vi "ReadData4.vi"() -> ()   [LabVIEW 2013]
uses:
  <vilib>/Utility/file.llb/Read From Spreadsheet File (DBL).vi
  <vilib>/Analysis/NI_AALPro.lvlib
  <vilib>/Analysis/NI_AALBase.lvlib
panel:
  out "Residual (V)":dbl=0.0015783758566444736 format="%#_3g"
  in  "1st sweep":i32=400
  out "Peak Area Distribution":cluster{"Y":dbl[], "Y":dbl[]}[](graph)
  in  "# of sweeps":i32=500
  out "Mean Error":dbl=-0.0 format="%#_2g"
  out "Mean Area":dbl=nan format="%#_4g"
  out "Peak Area":dbl(graph)=0.01758465336266432
  out "Spectrum #":i32=99
  out "Chars":i32=127116
  out "Fcen":dbl=213.0 format="%#_13g"
  out "Fmin":dbl=212.75 format="%#_13g"
  out "Fmax":dbl=213.25 format="%#_13g"
  out "# Data points":i32=101
  out "Peak Area (V-MHz)":dbl=0.01758465336266432 format="%#_3g"
  out "Offset V":dbl=0.15883666666666665 format="%#_3g"
  out "RMS Fit Error (V)":dbl=0.02098351608245331 format="%#_2g"
  in  "Start sigma (V)":dbl=0.01 format="%#_13g"
  in  "Start offset (V)":dbl format="%#_13g"
  out "FWHM (MHz)":dbl=0.06356226437922968 format="%#_3g"
  out "Center Freq (MHz)":dbl=213.00605703700742
  out "Amplitude (V)":dbl=0.2594313715946598 format="%#_3g"
  out "NMR Graph + Fit":cluster{cluster{dbl, "Numeric":dbl}[]}[](graph)=[{[{212.75, "Numeric"=0.0015783758566444736}, {212.755, "Numeric"=0.0015783758566444736}, {212.76, "Numeric"=0.0015783758566444738}, {212.765, "Numeric"=0.001578375856644475}, {212.77, "Numeric"=0.0015783758566444812}, {212.775, "Numeric"=0.0015783758566445105}, {212.78, "Numeric"=0.0015783758566446499}, {212.785, "Numeric"=0.0015783758566452857}, {212.79, "Numeric"=0.0015783758566480905}, {212.795, "Numeric"=0.0015783758566600408}, {212.8, "Numeric"=0.0015783758567092245}, {212.805, "Numeric"=0.001578375856904754}, {212.81, "Numeric"=0.0015783758576555789}, {212.815, "Numeric"=0.0015783758604403309}, {212.82, "Numeric"=0.0015783758704160137}, {212.825, "Numeric"=0.0015783759049296919}, {212.83, "Numeric"=0.0015783760202526297}, {212.835, "Numeric"=0.0015783763923853246}, {212.84, "Numeric"=0.0015783775520111368}, {212.845, "Numeric"=0.0015783810414393363}, {212.85, "Numeric"=0.001578391180165903}, {212.855, "Numeric"=0.0015784196234293983}, {212.86, "Numeric"=0.0015784966629971626}, {212.865, "Numeric"=0.0015786981074140884}, {212.87, "Numeric"=0.0015792065815228248}, {212.875, "Numeric"=0.0015804454238471377}, {212.88, "Numeric"=0.0015833585127361727}, {212.885, "Numeric"=0.0015899690039745432}, {212.89, "Numeric"=0.001604443445366001}, {212.895, "Numeric"=0.0016350205758822818}, {212.9, "Numeric"=0.0016973293113763314}, {212.905, "Numeric"=0.0018197850215321532}, {212.91, "Numeric"=0.002051842634218605}, {212.915, "Numeric"=0.002475772272221433}, {212.92, "Numeric"=0.0032221351201092673}, {212.925, "Numeric"=0.004488095587701443}, {212.93, "Numeric"=0.006556012234299915}, {212.935, "Numeric"=0.009807511846233161}, {212.94, "Numeric"=0.014725912011117679}, {212.945, "Numeric"=0.021878260555252972}, {212.95, "Numeric"=0.03186855427769141}, {212.955, "Numeric"=0.04525702061056377}, {212.96, "Numeric"=0.06244728812435715}, {212.965, "Numeric"=0.08355329369325902}, {212.97, "Numeric"=0.10826881484354303}, {212.975, "Numeric"=0.13577113329731721}, {212.98, "Numeric"=0.16469255499354238}, {212.985, "Numeric"=0.19318627788517476}, {212.99, "Numeric"=0.2190958639769093}, {212.995, "Numeric"=0.24021330175604594}, {213.0, "Numeric"=0.25458558472826925}, {213.005, "Numeric"=0.26081171148423077}, {213.01, "Numeric"=0.25826773368606104}, {213.015, "Numeric"=0.24720980881335808}, {213.02, "Numeric"=0.2287316929031936}, {213.025, "Numeric"=0.2045864387749786}, {213.03, "Numeric"=0.1769125428292504}, {213.035, "Numeric"=0.14792371126304468}, {213.04, "Numeric"=0.11962410451484337}, {213.045, "Numeric"=0.09359805892361928}, {213.05, "Numeric"=0.070900243041303}, {213.055, "Numeric"=0.05204669417618943}, {213.06, "Numeric"=0.03708639769050977}, {213.065, "Numeric"=0.025721484339133512}, {213.07, "Numeric"=0.01744260434522061}, {213.075, "Numeric"=0.011652418610937937}, {213.08, "Numeric"=0.007760641839252166}, {213.085, "Numeric"=0.005244867041899054}, {213.09, "Numeric"=0.0036797949184575744}, {213.095, "Numeric"=0.002742324323160648}, {213.1, "Numeric"=0.0022014129453304474}, {213.105, "Numeric"=0.0019006705177802116}, {213.11, "Numeric"=0.0017394965734230348}, {213.115, "Numeric"=0.001656216913191255}, {213.12, "Numeric"=0.0016147192204692693}, {213.125, "Numeric"=0.0015947742229850028}, {213.13, "Numeric"=0.001585526335222514}, {213.135, "Numeric"=0.0015813890617758935}, {213.14, "Numeric"=0.0015796029605821915}, {213.145, "Numeric"=0.0015788587965180057}, {213.15, "Numeric"=0.0015785595374779014}, {213.155, "Numeric"=0.0015784433706199186}, {213.16, "Numeric"=0.0015783998384890756}, {213.165, "Numeric"=0.0015783840891219372}, {213.17, "Numeric"=0.00157837858774433}, {213.175, "Numeric"=0.0015783767322402767}, {213.18, "Numeric"=0.0015783761279313756}, {213.185, "Numeric"=0.0015783759378738358}, {213.19, "Numeric"=0.001578375880149261}, {213.195, "Numeric"=0.0015783758632173985}, {213.2, "Numeric"=0.001578375858420789}, {213.205, "Numeric"=0.001578375857108391}, {213.21, "Numeric"=0.0015783758567615637}, {213.215, "Numeric"=0.0015783758566730336}, {213.22, "Numeric"=0.0015783758566512058}, {213.225, "Numeric"=0.001578375856646007}, {213.23, "Numeric"=0.0015783758566448112}, {213.235, "Numeric"=0.0015783758566445454}, {213.24, "Numeric"=0.0015783758566444883}, {213.245, "Numeric"=0.0015783758566444766}, {213.25, "Numeric"=0.0015783758566444742}]}, {[{212.75, "Numeric"=0.031063080700891782}, {212.755, "Numeric"=0.02864126124269653}, {212.76, "Numeric"=-0.016894595611743196}, {212.765, "Numeric"=0.029517619934582878}, {212.77, "Numeric"=-0.025551934372606694}, {212.775, "Numeric"=-0.008125528238406676}, {212.78, "Numeric"=-0.002418306493811001}, {212.785, "Numeric"=-0.027438710682556017}, {212.79, "Numeric"=0.0020111238944827414}, {212.795, "Numeric"=-0.03626500577548768}, {212.8, "Numeric"=0.011442277348240076}, {212.805, "Numeric"=-0.0496524014436506}, {212.81, "Numeric"=-0.03692948119914727}, {212.815, "Numeric"=0.0012352401786166756}, {212.82, "Numeric"=-0.03602967159264306}, {212.825, "Numeric"=0.01760845127854463}, {212.83, "Numeric"=-0.0448138678705418}, {212.835, "Numeric"=0.013143517432053747}, {212.84, "Numeric"=0.0051241576469458205}, {212.845, "Numeric"=-0.011825199458837116}, {212.85, "Numeric"=0.013245196212146149}, {212.855, "Numeric"=-0.028212086895564703}, {212.86, "Numeric"=0.004858164345331262}, {212.865, "Numeric"=-0.03808635623616108}, {212.87, "Numeric"=0.028614370992108368}, {212.875, "Numeric"=0.00042254508276021174}, {212.88, "Numeric"=0.008102406105732235}, {212.885, "Numeric"=0.01672010421806569}, {212.89, "Numeric"=-0.009656424272778075}, {212.895, "Numeric"=0.025042425694142723}, {212.9, "Numeric"=-0.008112183353736091}, {212.905, "Numeric"=0.02375236299291253}, {212.91, "Numeric"=-0.02568996924334846}, {212.915, "Numeric"=0.04033604225333626}, {212.92, "Numeric"=0.003706785371929616}, {212.925, "Numeric"=0.006699727121910387}, {212.93, "Numeric"=0.03229333113172461}, {212.935, "Numeric"=0.002166978796247526}, {212.94, "Numeric"=0.04390089378450415}, {212.945, "Numeric"=0.008876069631273187}, {212.95, "Numeric"=0.061874200147450625}, {212.955, "Numeric"=0.006177612394387855}, {212.96, "Numeric"=0.0718692019767547}, {212.965, "Numeric"=0.08523237041712214}, {212.97, "Numeric"=0.09155096438282276}, {212.975, "Numeric"=0.1650092165426851}, {212.98, "Numeric"=0.16219168783705415}, {212.985, "Numeric"=0.21698321094974346}, {212.99, "Numeric"=0.18876883477489367}, {212.995, "Numeric"=0.25293376967554815}, {213.0, "Numeric"=0.23116333333333336}, {213.005, "Numeric"=0.25444289699111866}, {213.01, "Numeric"=0.26325783189177343}, {213.015, "Numeric"=0.22639345571692407}, {213.02, "Numeric"=0.24873497882961174}, {213.025, "Numeric"=0.20576745012398104}, {213.03, "Numeric"=0.21967570228384378}, {213.035, "Numeric"=0.12354429624954497}, {213.04, "Numeric"=0.14695746468991325}, {213.045, "Numeric"=0.0842990542722811}, {213.05, "Numeric"=0.06175246651921382}, {213.055, "Numeric"=0.04460059703539199}, {213.06, "Numeric"=0.00682577288216199}, {213.065, "Numeric"=0.028509687870419714}, {213.07, "Numeric"=-0.014566664465056028}, {213.075, "Numeric"=0.027176939544759693}, {213.08, "Numeric"=-0.013980118705266859}, {213.085, "Numeric"=0.0049406244133277655}, {213.09, "Numeric"=0.004516635910013944}, {213.095, "Numeric"=-0.009675696326245403}, {213.1, "Numeric"=0.005238850020405028}, {213.105, "Numeric"=-0.015065759027471676}, {213.11, "Numeric"=0.020883090939438798}, {213.115, "Numeric"=-0.021243437551403205}, {213.12, "Numeric"=0.012924260560932321}, {213.125, "Numeric"=-0.00524587841609353}, {213.13, "Numeric"=0.010012295674560717}, {213.135, "Numeric"=0.02196302290283267}, {213.14, "Numeric"=0.007468502321343051}, {213.145, "Numeric"=0.03098875356222547}, {213.15, "Numeric"=-0.011518529545482908}, {213.155, "Numeric"=0.024701866125503097}, {213.16, "Numeric"=0.009002509019723076}, {213.165, "Numeric"=0.00013314923461824058}, {213.17, "Numeric"=0.022240534537217}, {213.175, "Numeric"=0.007868215388114136}, {213.18, "Numeric"=0.02875633825930482}, {213.185, "Numeric"=-0.0013585735119516495}, {213.19, "Numeric"=0.0260561478658157}, {213.195, "Numeric"=0.009929068110322653}, {213.2, "Numeric"=0.0047843893184356945}, {213.205, "Numeric"=0.02254167244214414}, {213.21, "Numeric"=0.013915542772177297}, {213.215, "Numeric"=0.023915377349219807}, {213.22, "Numeric"=0.004744973160478699}, {213.225, "Numeric"=0.025502194905078435}, {213.23, "Numeric"=-0.02362139896071716}, {213.235, "Numeric"=0.00045904673207106117}, {213.24, "Numeric"=0.006421262278401146}, {213.245, "Numeric"=-0.025864594576034267}, {213.25, "Numeric"=0.0010635859657747992}]}]
  out "File size (bytes)":i32=1284000
  out "Waveform Array":dbl[](array[numeric])=[-0.1506, -0.121, -0.1368, -0.0628, -0.0923, -0.0512, -0.0236, -0.0284, 0.0197, -0.0014, 0.0621, 0.0155, 0.0415, 0.0918, 0.0656, 0.1293, 0.076, 0.1422, 0.1416, 0.1313, 0.1623, 0.1261, 0.1638, 0.1249, 0.1951, 0.1699, 0.1801, 0.1908, 0.1661, 0.2021, 0.1699, 0.2024, 0.1533, 0.2194, 0.1826, 0.1852, 0.2102, 0.1793, 0.2201, 0.184, 0.2358, 0.1788, 0.2431, 0.255, 0.2598, 0.3317, 0.3273, 0.3805, 0.3507, 0.4133, 0.39, 0.4118, 0.4192, 0.381, 0.4021, 0.358, 0.3709, 0.2739, 0.2966, 0.2334, 0.2105, 0.1932, 0.1555, 0.1775, 0.135, 0.1776, 0.1376, 0.158, 0.1594, 0.1474, 0.1649, 0.1476, 0.187, 0.1488, 0.1874, 0.1742, 0.195, 0.2131, 0.2054, 0.2364, 0.2021, 0.2473, 0.2414, 0.2432, 0.2769, 0.2751, 0.3096, 0.2942, 0.3375, 0.3385, 0.3518, 0.3894, 0.4021, 0.435, 0.4404, 0.4875, 0.4666, 0.5209, 0.5592, 0.5615, 0.6254]
  out "File name":string="C:\\Documents and Settings\\Patrick McGaughey\\Desktop\\rssmt\\NMR3489061581.xls"
  # "Gaussian Fit Results"
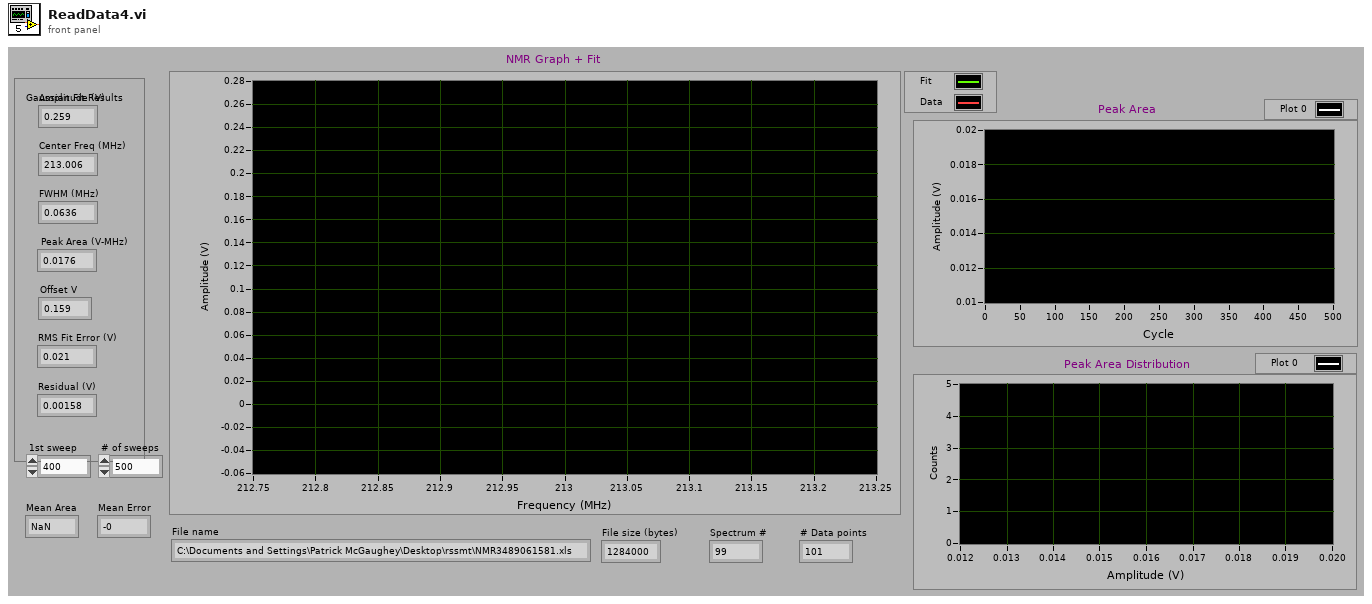
[diagram p1: front panel]
types:
  T1 = cluster{dbl, dbl, "Start sigma (V)":dbl, "Start offset (V)":dbl}
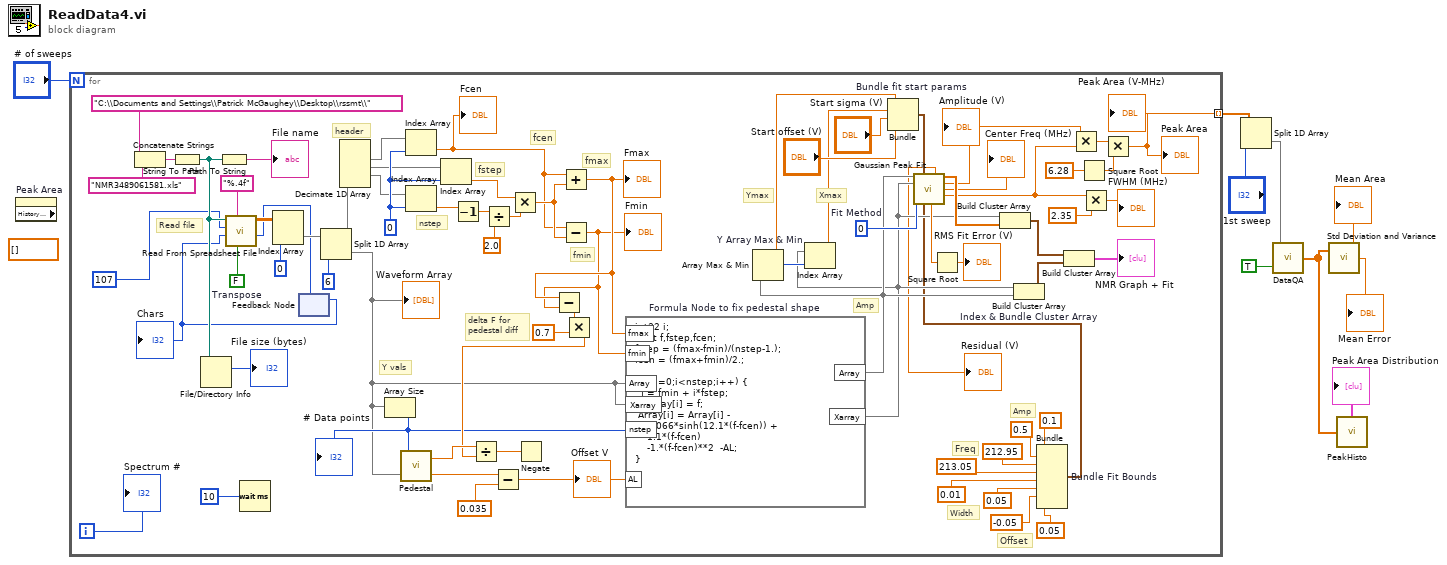
[diagram p0: block diagram]
diagram:
  (unwired) dbl[] []
  n1 = property on="Peak Area" class="WFChart (strict)" props=["History Data"]() -> ()  [unwired: 2 in, 3 out]
  n2 = for {
    N: "# of sweeps" -> [_]
    tunnel: [w23] -> w3 mode=indexing
    i -> [w24]
    w38 = 0
    w69 = 0  # Fit Method
    w80 = FALSE  # Transpose
    # "Amp"
    # "Offset"
    # "Width"
    # "Freq"
    # "Read file"
    # "header"
    # "nstep"
    # "fstep"
    # "fcen"
    # "fmin"
    # "fmax"
    # "Amp"
    # "delta F for\npedestal diff"
    # "Ymax"
    # "Xmax"
    # "Y vals"
    n3 = Concatenate Strings "Concatenate Strings"("C:\\Documents and Settings\\Patrick McGaughey\\Desktop\\rssmt\\", "NMR3489061581.xls") -> (w83:string)
    n4 = String To Path(string=w83) -> (path=w79:path)
    n5 = File/Directory Info(path=w79) -> (size=→"File size (bytes)":i64)  [unwired: 1 in, 6 out]
    n6 = Path To String(path=w79) -> (string=→"File name":string)
    n7 = Wait (ms)(milliseconds to wait=10) -> ()  [unwired: 1 out]
    n8 = feedback #1() -> (w25:i32)  [unwired: 1 in]
    "Chars" <- w25
    n9 = call-poly <vilib>:"Read From Spreadsheet File.vi"("transpose (no:F)"=w80, "format (%.3f)"="%.4f", "start of read offset (chars.:0)"=w25, "number of rows (all:-1)"=107, "file path (dialog if empty)"=w79) -> ("mark after read (chars.)"=w26:i32, "all rows"=w46:dbl[][])  [unwired: 2 in, 3 out]
    n10 = Index Array "Index Array"(array=w46, index (col)=0) -> (element=w44:dbl[])  [unwired: 1 in]
    n11 = feedback-in #1(w26) -> ()
    n12 = Split 1D Array(array=w44, index=6) -> (first subarray=w47:dbl[], second subarray=w31:dbl[])
    "Waveform Array" <- w31
    n13 = Decimate 1D Array(w47) -> (w39:dbl[], w37:dbl[], w36:dbl[])  [unwired: 3 out]
    n14 = Array Size(array=w31) -> (size(s)=w49:i32)
    "# Data points" <- w49
    n15 = call "Pedestal.vi"("Varray"=w31, "ArraySize"=w49) -> ("Average"=w11:dbl, "L-R"=w62:dbl)
    n16 = Index Array "Index Array"(array=w39, index=w38) -> (element=w27:dbl)
    "Fcen" <- w27
    n17 = Index Array(array=w36, index=w38) -> (element=w34:dbl)
    n18 = Index Array(array=w37, index=w38) -> (element=w35:dbl)
    n19 = Decrement(x=w34) -> (x-1=w43:dbl)
    n20 = Divide(x=w43, y=2.0) -> (x/y=w41:dbl)
    n21 = Subtract(x=w11, y=0.035) -> (x-y=w10:dbl)
    "Offset V" <- w10
    n22 = Multiply(x=w35, y=w41) -> (x*y=w40:dbl)
    n23 = Add(x=w27, y=w40) -> (x+y=w33:dbl)
    "Fmax" <- w33
    n24 = Subtract(x=w27, y=w40) -> (x-y=w32:dbl)
    "Fmin" <- w32
    n25 = Subtract(x=w33, y=w32) -> (x-y=w60:dbl)
    n26 = Multiply(x=w60, y=0.7) -> (x*y=w59:dbl)
    n27 = Divide(x=w62, y=w59) -> (x/y=w58:dbl)
    n28 = Negate(x=w58) -> ()  [unwired: 1 out]
    n29 = formula code="int32 i;\nfloat f,fstep,fcen;\nfstep = (fmax-fmin)/(nstep-1.);\nfcen = (fmax+fmin)/2.;\n\nfor (i=0;i<nstep;i++) {\n  f = fmin + i*fstep;\n  Xarray[i] = f;\n Array[i] = Array[i] - \n    0.066*sinh(12.1*(f-fcen)) +\n    1.1*(f-fcen)  \n    -1.*(f-fcen)**2  -AL;\n}" "Formula Node to fix pedestal shape"("nstep"=w49, "fmin"=w32, "fmax"=w33, "AL"=w10, "Array"=w31, "Xarray"=w31) -> ("Array"=w51:dbl[], "Xarray"=w50:dbl[])
    n30 = Array Max & Min "Y Array Max & Min"(array=w51) -> (max value=w68:dbl, max index (indices)=w67:i32)  [unwired: 2 out]
    n31 = Index Array "Index Array"(array=w50, index=w67) -> (element=w55:dbl)
    n32 = Bundle "Bundle fit start params"(w68, w55, "Start sigma (V)"="Start sigma (V)", "Start offset (V)"="Start offset (V)") -> (w74:T1)  [unwired: 1 in]
    n33 = Build Cluster Array "Index & Bundle Cluster Array"(w50, w51) -> (w73:cluster{dbl, dbl}[])
    n34 = Bundle "Bundle Fit Bounds"(0.1, 0.5, 212.95, 213.05, 0.01, 0.05, -0.05, 0.05) -> (w13:cluster{dbl, dbl, dbl, dbl, dbl, dbl, dbl, dbl})  [unwired: 1 in]
    n35 = call <vilib>:"Gaussian Peak Fit.vi"("Y"=w51, "initial guess"=w74, "X"=w50, "method"=w69, "parameter bounds"=w13) -> ("offset"=→"Residual (V)":dbl, "Best Gaussian Fit"=w77:dbl[], "amplitude"=w66:dbl, "center"=→"Center Freq (MHz)":dbl, "standard deviation"=w54:dbl, "residue"=w57:dbl)  [unwired: 4 in, 1 out]
    "Amplitude (V)" <- w66
    n36 = Square Root(x=w57) -> (sqrt(x)=→"RMS Fit Error (V)":dbl)
    n37 = Build Cluster Array ("Index & Bundle Cluster Array")(w50, w77) -> (w30:cluster{dbl, "Numeric":dbl}[])
    n38 = Build Cluster Array "Build Cluster Array"(w30, w73) -> (→"NMR Graph + Fit":cluster{cluster{dbl, "Numeric":dbl}[]}[])
    n39 = Multiply(x=w66, y=w54) -> (x*y=w63:dbl)
    n40 = Square Root(x=6.28) -> (sqrt(x)=w64:dbl)
    n41 = Multiply(x=w54, y=2.35) -> (x*y=→"FWHM (MHz)":dbl)
    n42 = Multiply(x=w63, y=w64) -> (x*y=w23:dbl)
    "Peak Area (V-MHz)" <- w23
    "Peak Area" <- w23
    "Spectrum #" <- w24
  }
  n43 = Split 1D Array(array=w3, index="1st sweep") -> (second subarray=w1:dbl[])  [unwired: 1 out]
  n44 = call "DataQA.vi"("Quality cuts"=TRUE, "Data In"=w1) -> ("Data Out"=w4:dbl[])
  n45 = call <vilib>:"Std Deviation and Variance.vi"("X"=w4) -> ("mean"=→"Mean Area":dbl, "standard deviation"=→"Mean Error":dbl)  [unwired: 1 in, 1 out]
  n46 = call "PeakHisto.vi"("Data Out"=w4) -> ("XY Graph"=→"Peak Area Distribution":cluster{"Y":dbl[], "Y":dbl[]}[])
